vi "Font Read.vi"(4 "error in (no error)":errorcluster, 6 "Container State":T4, 7 "Display State In":T1) -> (0 "error out":errorcluster, 2 "Value":T3, 3 "Display State Out":T1)   [LabVIEW 2012, in "Hover Button.xctl"]
uses:
  Hover Button.xctl
  <vilib>/_xctls/Container State.ctl
  Font Properties.ctl
  State.ctl
  Button Colors.ctl
  <vilib>/_xctls/XControlSupport.lvlib
panel:
  # "Replace the Value Indicator below with an Indicator of desired type.\nDo not remove this Indicator or the others from the connector pane. \nDo not change the connector pane pattern.\nThe Value Indicator should always be the second terminal from top on the output side in the connector pane."
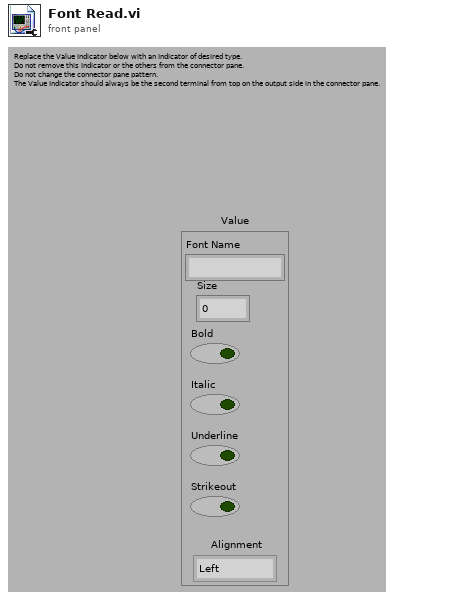
[diagram p1: front panel]
types:
  T1 = typedef "Hover Button.xctl/State.ctl" = cluster{"On Text":string, "Off Text":string, "Current Color":T2, "Button Color":T2, "Hover Color":T2, "Show Boolean Text":bool, "Multiple Strings":bool, "Font":T3}
  T2 = typedef "Hover Button.xctl/Button Colors.ctl" = cluster{"On Color":u32, "Text Color":u32, "Off Color":u32}
  T3 = typedef "Hover Button.xctl/Font Properties.ctl" = cluster{"Font Name":string, "Size":u32, "Bold":bool, "Italic":bool, "Underline":bool, "Strikeout":bool, "Alignment":enum16{"Left", "Center", "Right"}}
  T4 = typedef "XControlSupport.lvlib/Container State.ctl" = cluster{"Indicator?":bool, "Run Mode?":bool, " Refnum":refnum<vi>}
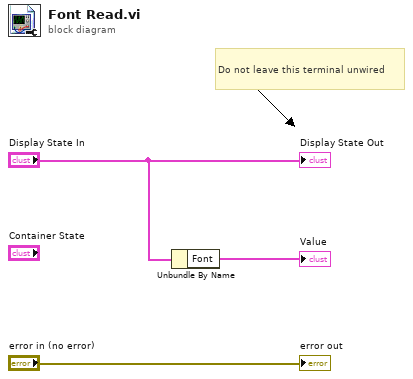
[diagram p0: block diagram]
diagram:
  # "Do not leave this terminal unwired"
  n1 = Unbundle By Name("Display State In") -> ("Font"=→"Value":T3)
  "error out" <- "error in (no error)"
  "Display State Out" <- "Display State In"
